vi "Extract Tip.vi"(6 "Label":string, 8 "error in (no error)":errorcluster, 9 "Tip Number":i32, 10 "Tip":T2={"Point"={"X"=0.0, "Y"=0.0}, "Angle"=0.0, "Frame Number"=0, "ROI Descriptor"={"Global Rectangle"=[], "Contours"=[]}, "Curvature"=0.0, "Label"="Non-tip"} {"ROI Descriptor"."Contours"."Type" items=["No Selection", "Point", "Line", "Rectangle", "Oval", "Polygon", "Freehand Region", "Annulus", "Unused2", "Unused3", "Broken Line", "Freehand Line", "Rotated Rectangle"]; "Point"."Y" format="%.2f"; "Point"."X" format="%.2f"}, 11 "Image Array":T1[](array[typedef])) -> (0 "error out":errorcluster, 3 "Tip Image":T1)   [LabVIEW 2013]
uses:
  <vilib>/vision/Image Controls.llb/IMAQ Image.ctl
  Controls/Tip.ctl
  <vilib>/vision/NI_Vision_Development_Module.lvlib
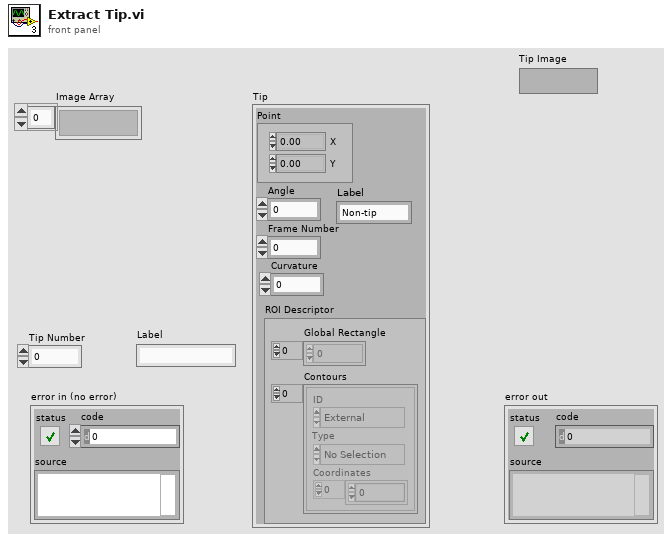
[diagram p1: front panel]
types:
  T1 = typedef "IMAQ Image.ctl" = refnum<image>
  T2 = typedef "Tip.ctl" = cluster{"Point":T3, "Angle":dbl, "Frame Number":i32, "ROI Descriptor":T4, "Curvature":dbl, "Label":string}
  T3 = typedef "IMAQ Point" = cluster{"X":sgl, "Y":sgl}
  T4 = typedef "ROI Descriptor" = cluster{"Global Rectangle":i32[], "Contours":cluster{"ID":enum32{"External", "Internal"}, "Type":u32, "Coordinates":i32[]}[]}
  T5 = typedef "Image Type" = u32
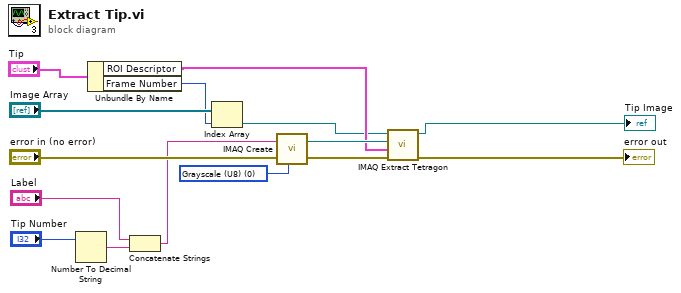
[diagram p0: block diagram]
diagram:
  w11 = T5 0 items=["Grayscale (U8)", "Grayscale (I16)", "Grayscale (SGL)", "Complex (CSG)", "RGB (U32)", "HSL (U32)", "RGB (U64)", "Grayscale (U16)"] ("Image Type")
  n1 = Number To Decimal String(number="Tip Number") -> (decimal integer string=w13:string)  [unwired: 1 in]
  n2 = Unbundle By Name("Tip") -> ("ROI Descriptor"=w4:T4, "Frame Number"=w2:i32)
  n3 = Concatenate Strings("Label", w13) -> (w12:string)
  n4 = Index Array(array="Image Array", index=w2) -> (element=w1:T1)
  n5 = call "IMAQ Create"("Image Name"=w12, "Image Type"=w11, "error in (no error)"="error in (no error)") -> ("New Image"=w8:T1, "error out"=w9:errorcluster)  [unwired: 2 in]
  n6 = call-poly "IMAQ Extract Tetragon"("error in (no error)"=w9, "ROI Descriptor"=w4, "Image Dst"=w8, "Image Src"=w1) -> ("error out"=→"error out":errorcluster, "Image Dst Out"=→"Tip Image":T1)  [unwired: 6 in]
